vi "Tool OpCfg Parse from GXML String.vi"(8 "error in (no error)":errorcluster, 11 "XML String In":string) -> (0 "error out":errorcluster, 3 "Tool Op Cfg Cluster out":T1={"Use Tool Cfg"=FALSE, "Use Tool Cal"=FALSE, "Fake Data?"=FALSE, "Mode"=-2, "Array Subset Length"=30, "nArrays to Read"=2, "Full Array Read Length"=500, "nSubarrays/Sensor"=0})   [LabVIEW 2015, in "Tool Cfg.lvlib"]
uses:
  Tool Cfg.lvlib
  _Tool Operation Config Cluster--typedef.ctl
  _Tool OpCfg GXML Format Cluster--typedef.ctl
  <vilib>/NI/GXML/_subVIs/GXML SearchParser/Search Parser.vi
  <vilib>/NI/GXML/GXML.lvlib
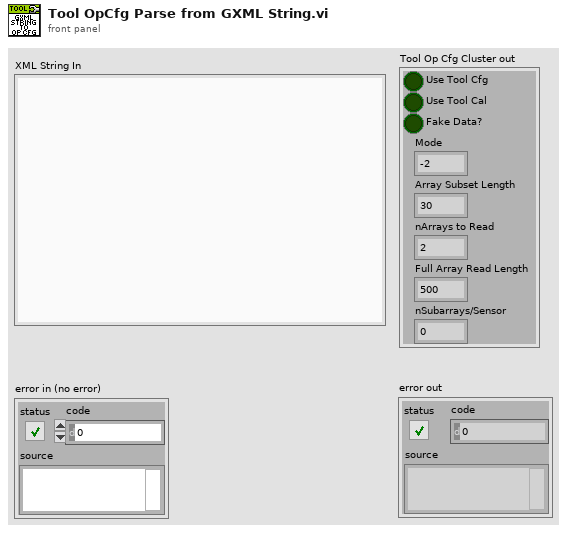
[diagram p1: front panel]
types:
  T1 = typedef "Tool Cfg.lvlib/_Tool Operation Config Cluster--typedef.ctl" = cluster{"Use Tool Cfg":bool, "Use Tool Cal":bool, "Fake Data?":bool, "Mode":i16, "Array Subset Length":i16, "nArrays to Read":i16, "Full Array Read Length":i16, "nSubarrays/Sensor":i16}
  T2 = typedef "Tool Cfg.lvlib/_Tool OpCfg GXML Format Cluster--typedef.ctl" = cluster{"Use Tool Cfg":bool, "Use Tool Cal":bool, "Fake Data":bool, "Mode":i16, "Array Subset Length":i16, "nArrays to Read":i16, "Full Array Read Length":i16, "nSubarraysPerSensor":i16}
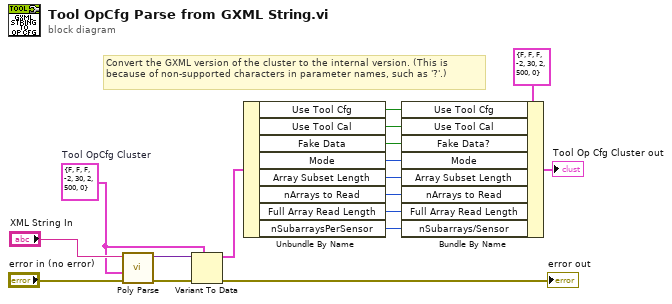
[diagram p0: block diagram]
diagram:
  w14 = T2 {"Use Tool Cfg"=FALSE, "Use Tool Cal"=FALSE, "Fake Data"=FALSE, "Mode"=-2, "Array Subset Length"=30, "nArrays to Read"=2, "Full Array Read Length"=500, "nSubarraysPerSensor"=0}  # Tool OpCfg Cluster
  # "Convert the GXML version of the cluster to the internal version. (This is because of non-supported characters in parameter names, such as '?'.)"
  n1 = call-poly <vilib>:"Poly Parse.vi"("error in"="error in (no error)", "TypeDesc"=w14, "XML String In"="XML String In") -> ("error out"=w15:errorcluster, "Parsed Data"=w16:variant)  [unwired: 7 in]
  n2 = Variant To Data(error in=w15, type=w14, Variant=w16) -> (data=w12:T2, error out=→"error out":errorcluster)
  n3 = Unbundle By Name(w12) -> ("Use Tool Cfg"=w11:bool, "Use Tool Cal"=w10:bool, "Fake Data"=w9:bool, "Mode"=w8:i16, "Array Subset Length"=w7:i16, "nArrays to Read"=w6:i16, "Full Array Read Length"=w5:i16, "nSubarraysPerSensor"=w4:i16)
  n4 = Bundle By Name(cluster=T1 {"Use Tool Cfg"=FALSE, "Use Tool Cal"=FALSE, "Fake Data?"=FALSE, "Mode"=-2, "Array Subset Length"=30, "nArrays to Read"=2, "Full Array Read Length"=500, "nSubarrays/Sensor"=0} ("Tool Operation Config"), "Use Tool Cfg"=w11, "Use Tool Cal"=w10, "Fake Data?"=w9, "Mode"=w8, "Array Subset Length"=w7, "nArrays to Read"=w6, "Full Array Read Length"=w5, "nSubarrays/Sensor"=w4) -> (→"Tool Op Cfg Cluster out":T1)
